vi "set_target.vi"(2 "error in (no error)":errorcluster, 3 "Remote Server Address":string="palantir", 4 "CommonTargetData":T1) -> (0 "error out":errorcluster, 1 "success":bool)   [LabVIEW 2011]
uses:
  TCPdata.ctl
  TargetData.ctl
  CommonTargetData.ctl
panel:
  in  "Cluster":T2
  in  "Listen Port":u16=5311
  in  "Remote Server Port":u16=5310
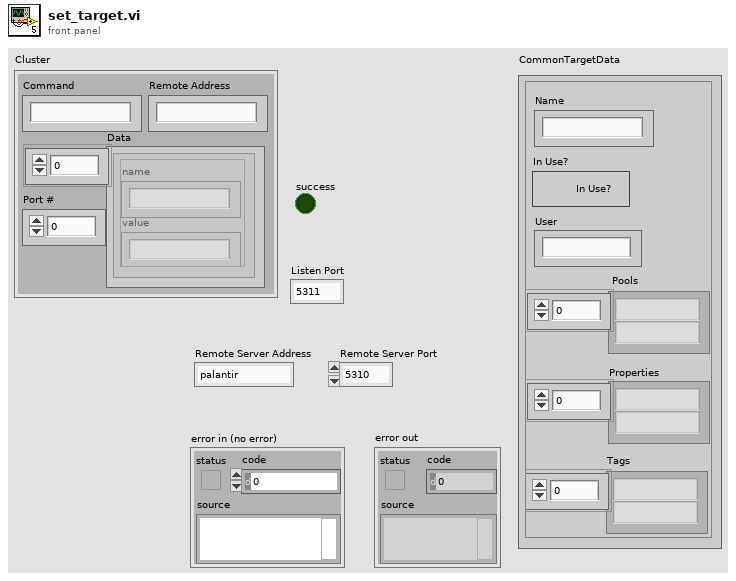
[diagram p1: front panel]
types:
  T1 = typedef "CommonTargetData.ctl" = cluster{"Name":string, "In Use?":bool, "User":string, " Pools":string[], "Tags":string[], "Properties":string[]}
  T2 = typedef "TCPdata.ctl" = cluster{"Data":T3, "Command":string, "Remote Address":string, "Port #":u16}
  T3 = typedef "TargetData.ctl" = cluster{"name":string, "value":string}[]
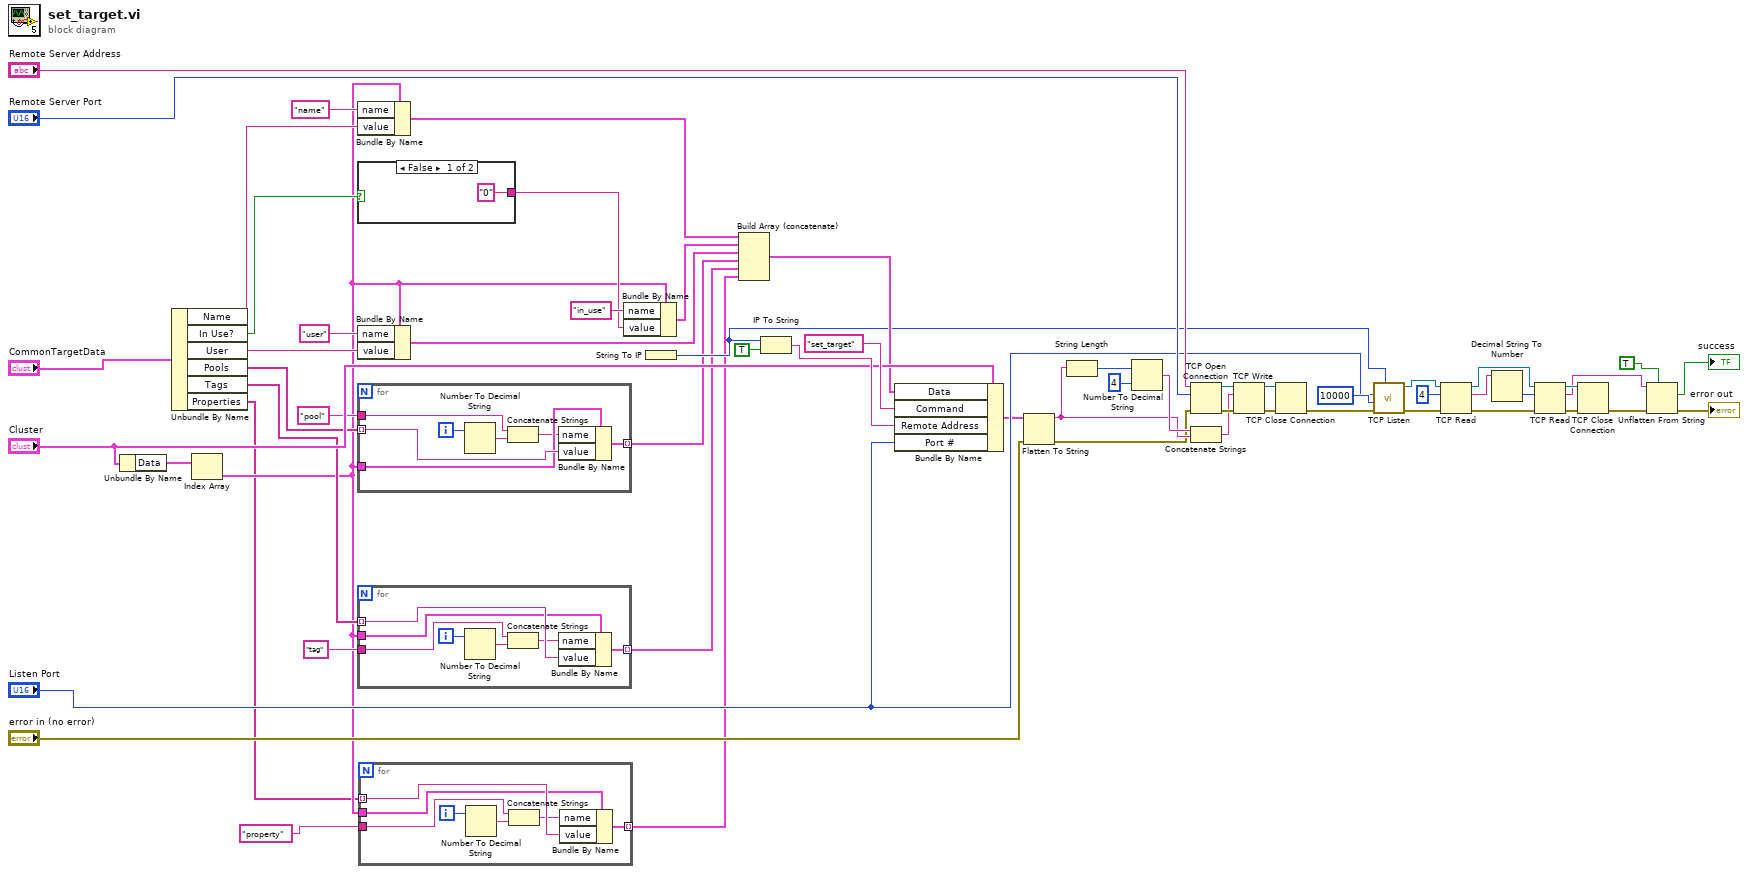
[diagram p0: block diagram]
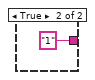
[diagram p2: hidden frame]
diagram:
  n1 = Unbundle By Name("Cluster") -> ("Data"=w44:T3)
  n2 = Unbundle By Name("CommonTargetData") -> ("Name"=w13:string, "In Use?"=w12:bool, "User"=w11:string, "Pools"=w9:string[], "Tags"=w6:string[], "Properties"=w1:string[])
  n3 = Index Array(array=w44) -> (element=w2:cluster{"name":string, "value":string})  [unwired: 1 in]
  n4 = Bundle By Name(cluster=w2, "name"="name", "value"=w13) -> (w43:cluster{"name":string, "value":string})
  n5 = case shown="False" w12 {
    tunnel: ["0" ("value") "1" ("value")] -> w15
    frame False {
    }
    frame True {
    }
  }
  n6 = Bundle By Name(cluster=w2, "name"="user", "value"=w11) -> (w16:cluster{"name":string, "value":string})
  n7 = for {
    tunnel: "pool" ("name") -> [w66]
    tunnel: w9 -> [w68] mode=indexing
    tunnel: w2 -> [w67]
    tunnel: [w62] -> w8 mode=indexing
    i -> [w65]
    n8 = Number To Decimal String(number=w65) -> (decimal integer string=w64:string)  [unwired: 1 in]
    n9 = Concatenate Strings(w66, w64) -> (w63:string)
    n10 = Bundle By Name(cluster=w67, "name"=w63, "value"=w68) -> (w62:cluster{"name":string, "value":string})
  }
  n11 = for {
    tunnel: "tag" ("name") -> [w73]
    tunnel: w6 -> [w75] mode=indexing
    tunnel: w2 -> [w74]
    tunnel: [w69] -> w5 mode=indexing
    i -> [w72]
    n12 = Number To Decimal String(number=w72) -> (decimal integer string=w71:string)  [unwired: 1 in]
    n13 = Concatenate Strings(w73, w71) -> (w70:string)
    n14 = Bundle By Name(cluster=w74, "name"=w70, "value"=w75) -> (w69:cluster{"name":string, "value":string})
  }
  n15 = for {
    tunnel: "property" ("name") -> [w80]
    tunnel: w1 -> [w82] mode=indexing
    tunnel: w2 -> [w81]
    tunnel: [w76] -> w3 mode=indexing
    i -> [w79]
    n16 = Number To Decimal String(number=w79) -> (decimal integer string=w78:string)  [unwired: 1 in]
    n17 = Concatenate Strings(w80, w78) -> (w77:string)
    n18 = Bundle By Name(cluster=w81, "name"=w77, "value"=w82) -> (w76:cluster{"name":string, "value":string})
  }
  n19 = Bundle By Name(cluster=w2, "name"="in_use", "value"=w15) -> (w17:cluster{"name":string, "value":string})
  n20 = String To IP() -> (0:w40:u32)  [unwired: 1 in]
  n21 = Build Array (concatenate)(w43, w17, w16, w8, w5, w3) -> (w42:cluster{"name":string, "value":string}[])
  n22 = IP To String(1:TRUE ("dot notation? (F)"), 2:w40) -> (0:w47:string)
  n23 = Bundle By Name(cluster="Cluster", "Data"=w42, "Command"="set_target", "Remote Address"=w47, "Port #"="Listen Port") -> (w35:T2)
  n24 = Flatten To String(anything=w35, error in (no error)="error in (no error)") -> (data string=w34:string, error out=w32:errorcluster)  [unwired: 2 in, 1 out]
  n25 = String Length(string=w34) -> (length=w38:i32)
  n26 = Number To Decimal String(number=w38, width (-)=i16 4) -> (decimal integer string=w37:string)
  n27 = TCP Open Connection(address="Remote Server Address", remote port or service name="Remote Server Port", error in (no error)=w32) -> (connection ID=w59:refnum<k5>, error out=w58:errorcluster)  [unwired: 2 out]
  n28 = Concatenate Strings(w37, w34) -> (w39:string)
  n29 = TCP Write(connection ID=w59, data in=w39, error in (no error)=w58) -> (connection ID out=w56:refnum<k5>, error out=w57:errorcluster)  [unwired: 2 out]
  n30 = TCP Close Connection(connection ID=w56, error in (no error)=w57) -> (error out=w50:errorcluster)  [unwired: 2 out]
  n31 = call <vilib>:"TCP Listen.vi"("net address"=w40, "error in (no error)"=w50, "timeout ms (wait forever: -1)"=10000, "port"="Listen Port") -> ("error out"=w29:errorcluster, "connection ID"=w27:refnum<k5>)  [unwired: 3 in, 3 out]
  n32 = TCP Read(connection ID=w27, bytes to read=4, error in (no error)=w29) -> (connection ID out=w26:refnum<k5>, data out=w30:string, error out=w28:errorcluster)  [unwired: 1 in, 1 out]
  n33 = Decimal String To Number(string=w30) -> (number=w25:i32)  [unwired: 2 in, 1 out]
  n34 = TCP Read(connection ID=w26, bytes to read=w25, error in (no error)=w28) -> (connection ID out=w53:refnum<k5>, data out=w23:string, error out=w51:errorcluster)  [unwired: 1 in, 1 out]
  n35 = TCP Close Connection(connection ID=w53, error in (no error)=w51) -> (error out=w24:errorcluster)  [unwired: 2 out]
  n36 = Unflatten From String(type=TRUE, binary string=w23, error in (no error)=w24) -> (value=→"success":bool, error out=→"error out":errorcluster)  [unwired: 2 in, 1 out]
